vi "SMTP.vi"(0 "Carrier":T1(ring), 1 "Outgoing Mail Server (SMTP)":string="smtp.gmail.com", 2 "Email":string="ece144.smtp@gmail.com", 3 "Password":string="LabVIEW_Texting", 4 "Phone Number":string, 5 "error in (no error)":errorcluster, 6 "Subject":string="Testing SMTP", 7 "Body":string="This is to test the SMTP.", 9 "attachments":path[](array[path])) -> (19 "error out":errorcluster)   [LabVIEW 2020]
doc: "Sends a message to the specified Phone Number using the Email, Carrier and Mail Server provided. You can insert a Subject, Body and/or files such as an Image."
uses:
  <vilib>/smtpClient/Set Message Text.vi
  <vilib>/smtpClient/LabVIEWSMTPClient.lvlib
panel:
  in  "TLS":bool=TRUE
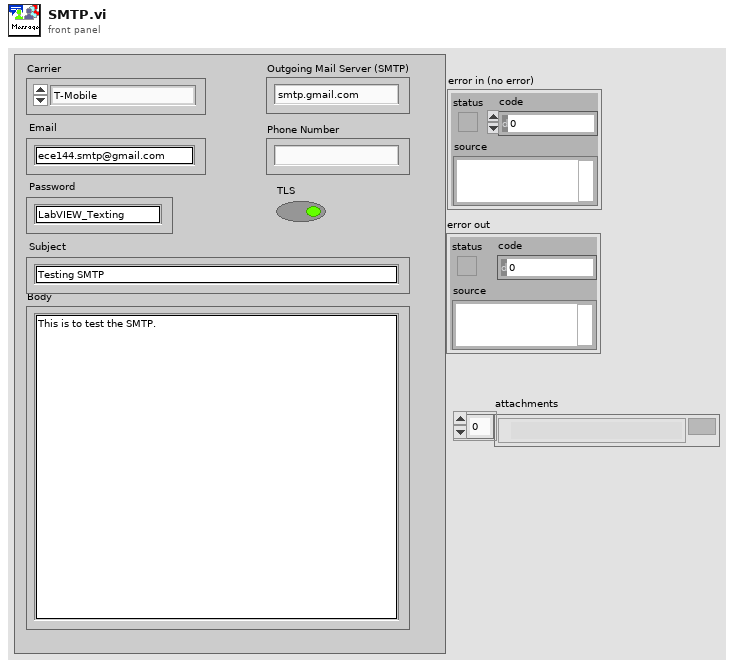
[diagram p1: front panel]
types:
  T1 = enum16{"T-Mobile", "AT&T", "Verizon", "Sprint", "Google-Fi"}
  T2 = typedef "LabVIEWSMTPClient.lvlib/SmtpClientHandle.ctl" = refnum<k1>
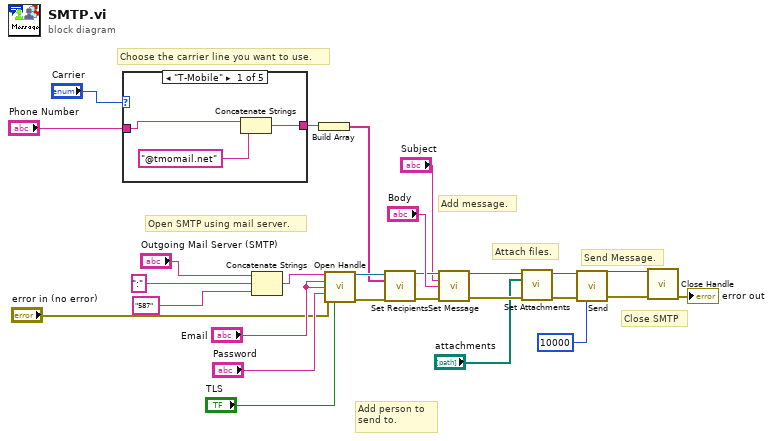
[diagram p0: block diagram]
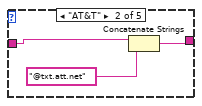
[diagram p2: hidden frame]
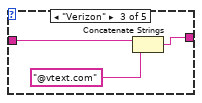
[diagram p3: hidden frame]
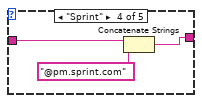
[diagram p4: hidden frame]
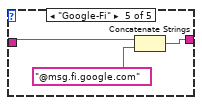
[diagram p5: hidden frame]
diagram:
  # "Attach files."
  # "Close SMTP"
  # "Send Message."
  # "Add message."
  # "Add person to \nsend to."
  # "Open SMTP using mail server."
  # "Choose the carrier line you want to use."
  n1 = case shown="\"T-Mobile\"" "Carrier" {
    tunnel: "Phone Number" -> [w29 w32 w35 w38 w40]
    tunnel: [w28 w31 w34 w37 w41] -> w17
    frame "T-Mobile" {
      n2 = Concatenate Strings(w29, "@tmomail.net") -> (w28:string)
    }
    frame "AT&T" {
      n3 = Concatenate Strings(w32, "@txt.att.net") -> (w31:string)
    }
    frame "Verizon" {
      n4 = Concatenate Strings(w35, "@vtext.com") -> (w34:string)
    }
    frame "Sprint" {
      n5 = Concatenate Strings(w38, "@pm.sprint.com") -> (w37:string)
    }
    frame "Google-Fi" {
      n6 = Concatenate Strings(w40, "@msg.fi.google.com") -> (w41:string)
    }
  }
  n7 = Concatenate Strings("Outgoing Mail Server (SMTP)", ":" ("string"), "587" ("string")) -> (w22:string)
  n8 = Build Array(w17) -> (w16:string[])
  n9 = call <vilib>:"Open Handle.vi"("server address"=w22, "from"="Email", "username"="Email", "password"="Password", "error in (no error)"="error in (no error)", "use TLS (false)"="TLS") -> ("handle out"=w18:T2, "error out"=w15:errorcluster)  [unwired: 8 in]
  n10 = call <vilib>:"Set Recipients.vi"("handle in"=w18, "to"=w16, "error in (no error)"=w15) -> ("handle out"=w13:T2, "error out"=w11:errorcluster)  [unwired: 11 in]
  n11 = call-poly <vilib>:"Set Message.vi"("handle in"=w13, "subject"="Subject", "plain text message"="Body", "error in (no error)"=w11) -> ("handle out"=w5:T2, "error out"=w4:errorcluster)  [unwired: 10 in]
  n12 = call <vilib>:"Set Attachments.vi"("handle in"=w5, "attachments"="attachments", "error in (no error)"=w4) -> ("handle out"=w1:T2, "error out"=w2:errorcluster)  [unwired: 11 in]
  n13 = call <vilib>:"Send.vi"("handle in"=w1, "error in (no error)"=w2, "timeout in ms (10000)"=10000) -> ("handle out"=w9:T2, "error out"=w8:errorcluster)  [unwired: 10 in, 1 out]
  n14 = call <vilib>:"Close Handle.vi"("handle in"=w9, "error in (no error)"=w8) -> ("error out"=→"error out":errorcluster)  [unwired: 12 in, 1 out]
